vi "Stop FP.vi"(8 "error in":errorcluster, 11 "Pcal GUI in":refnum<class "Pcal GUI.lvclass">) -> (0 "error out":errorcluster, 3 "Pcal GUI out":refnum<class "Pcal GUI.lvclass">)   [LabVIEW 2015, in "Pcal GUI.lvclass"]
uses:
  Pcal GUI.lvclass
  Pcal GUI.lvclass/Pcal GUI.ctl
  Reusable/GUI/GUI.lvclass
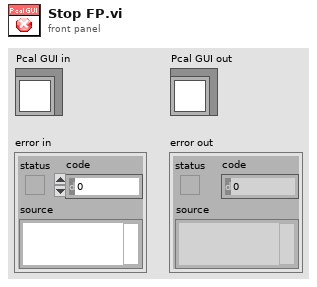
[diagram p1: front panel]
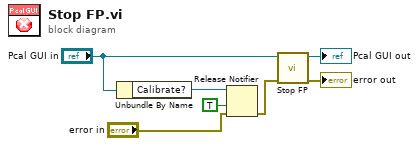
[diagram p0: block diagram]
diagram:
  n1 = Unbundle By Name("Pcal GUI in") -> ("Calibrate?"=w4:refnum<notifier>)
  n2 = Release Notifier(notifier=w4, force destroy? (F)=TRUE, error in (no error)="error in") -> (error out=w1:errorcluster)  [unwired: 2 out]
  n3 = call-parent "Stop FP.vi"("error in"=w1, "GUI in"="Pcal GUI in") -> ("error out"=→"error out":errorcluster, "GUI out"=→"Pcal GUI out":refnum<class "Pcal GUI.lvclass">)  [unwired: 8 in]
